vi "Read speed.vi"(7 "Simulate?":bool, 8 "error in (no error)":errorcluster, 11 "VISA Refnum in":refnum<visa-resource-name>) -> (0 "error out":errorcluster, 3 "number":dbl)   [LabVIEW 2020, in "Monochromator.lvlib"]
uses:
  Monochromator.lvlib
  <vilib>/Instr/_visa.llb/VISA Flush IO Buffer Mask.ctl
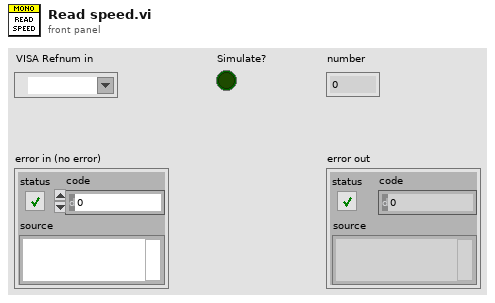
[diagram p1: front panel]
types:
  T1 = typedef "VISA Flush IO Buffer Mask.ctl" = u16
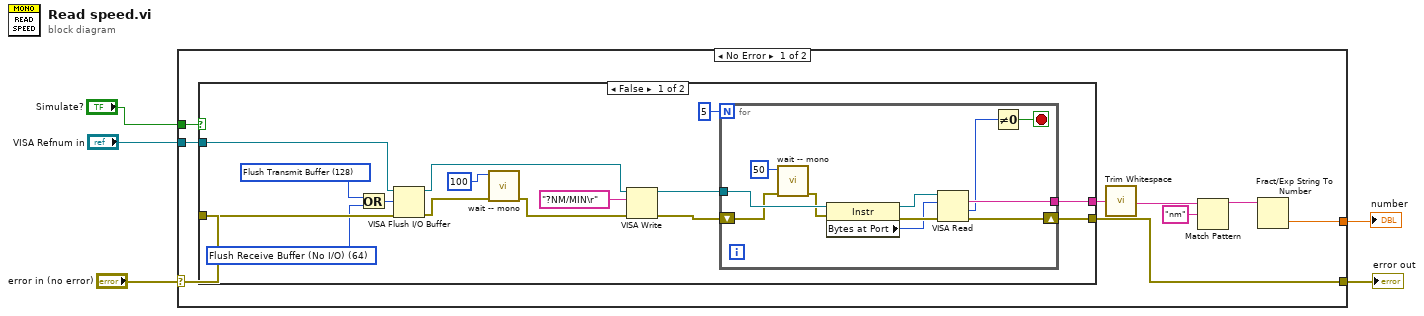
[diagram p0: block diagram]
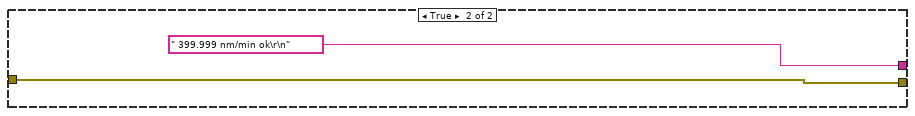
[diagram p2: hidden frame]
diagram:
  n1 = case shown="No Error" "error in (no error)" {
    selector: "error in (no error)" -> [w11 w43]
    tunnel: "VISA Refnum in" -> [w14 _]
    tunnel: [w10 w43] -> w3
    tunnel: "Simulate?" -> [w12 _]
    tunnel: [w6 _] -> w1
    frame No Error {
      n2 = case shown="False" w12 {
        tunnel: w14 -> [w23 _]
        tunnel: [w27 " 399.999 nm/min ok\r\n" ("read buffer")] -> w13
        tunnel: w11 -> [w24 w41]
        tunnel: [w26 w41] -> w10
        frame False {
          w17 = T1 64 items=["Flush Receive Buffer"=16, "Write Transmit Buffer to Device"=32, "Flush Receive Buffer (No I/O)"=64, "Flush Transmit Buffer"=128] ("Mask")
          w18 = T1 128 items=["Flush Receive Buffer"=16, "Write Transmit Buffer to Device"=32, "Flush Receive Buffer (No I/O)"=64, "Flush Transmit Buffer"=128] ("Mask")
          n3 = Or(x=w18, y=w17) -> (x .or. y?=w16:T1)
          n4 = VISA Flush I/O Buffer(VISA resource name=w23, mask (16)=w16, error in (no error)=w24) -> (VISA resource name out=w22:refnum<visa-resource-name>, error out=w21:errorcluster)
          n5 = call "wait -- mono.vi"("error in (no error)"=w21, "milliseconds to wait"=u32 100) -> ("error out"=w20:errorcluster)  [unwired: 9 in]
          n6 = VISA Write(VISA resource name=w22, write buffer="?NM/MIN\r", error in (no error)=w20) -> (VISA resource name out=w28:refnum<visa-resource-name>, error out=w25:errorcluster)  [unwired: 1 out]
          n7 = for {
            N: 5 -> [_]
            tunnel: w28 -> [w40]
            tunnel: [w36] -> w27
            shift-right: [w35] -> w26
            shift-left: w25 -> [w34]
            stop <- w30 stop-if-true
            n8 = call "wait -- mono.vi"("error in (no error)"=w34, "milliseconds to wait"=u32 50) -> ("error out"=w33:errorcluster)  [unwired: 9 in]
            n9 = property class="Instr"(reference=w40, error in=w33) -> (reference out=w38:refnum<visa-resource-name>, error out=w39:errorcluster, "Bytes at Port"=w37:u32)
            n10 = VISA Read(VISA resource name=w38, byte count=w37, error in (no error)=w39) -> (read buffer=w36:string, return count=w31:u32, error out=w35:errorcluster)  [unwired: 1 out]
            n11 = Not Equal To 0?(x=w31) -> (x != 0?=w30:bool)
          }
        }
        frame True {
        }
      }
      n12 = call <vilib>:"Trim Whitespace.vi"("string"=w13) -> ("trimmed string"=w9:string)  [unwired: 1 in]
      n13 = Match Pattern(string=w9, regular expression="nm") -> (before substring=w7:string)  [unwired: 1 in, 3 out]
      n14 = Fract/Exp String To Number(string=w7) -> (number=w6:dbl)  [unwired: 3 in, 1 out]
    }
    frame Error {
    }
  }
  "error out" <- w3
  "number" <- w1
